vi "Destroy Class ObjData.vi"(8 "error in (no error)":errorcluster, 11 "Motor Controller in":refnum<class "Motor Controller.lvclass">) -> (0 "error out":errorcluster, 3 "Motor Controller out":refnum<class "Motor Controller.lvclass">)   [LabVIEW 2022 SP3, in "Motor Controller.lvclass"]
uses:
  Motor Controller.lvclass
  Motor Controller.lvclass/Motor Controller.ctl
panel:
  out "ObjData Variant":variant
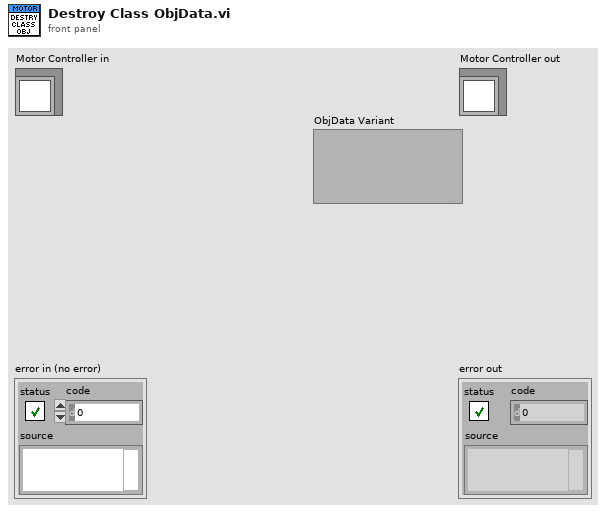
[diagram p1: front panel]
types:
  T1 = typedef "Motor Controller.lvclass/Private Data.ctl" = cluster{"UserEvents":T2, "All Dependencies":cluster{"Class References":refnum<class>[], "Class Names":string[]}, "Status":T3}
  T2 = typedef "Motor Controller.lvclass/UserEvents.ctl" = cluster{"API Incoming Event":refnum<user-event>, "API Executed Event":refnum<user-event>, "API Return Event":refnum<user-event>, "Status Changed Event":refnum<user-event>, "StopEvent":refnum<user-event>}
  T3 = typedef "Motor Controller.lvclass/Status.ctl" = cluster{"Motor Controller Config Data":T4, "Motor Controller Data":cluster{"Enabled?":bool}, "Stage Move":T5, "Stage Busy?":bool}
  T4 = typedef "Motor Controller.lvclass/Motor Controller Config Data.ctl" = cluster{"Motor IP Addresss":string, "Current Position":i32, "Pulse_Per_mm":i32, "PrePrint":dbl[], "Load Position_mm":i32, "Laminate Position_mm":i32}
  T5 = typedef "Motor Controller.lvclass/Stage Move Data.ctl" = cluster{"Current Step":string, "Move Data":T6[]}
  T6 = typedef "Motor Controller.lvclass/Batch Index Speed Data.ctl" = cluster{"Batch & Cycle":string, "Move":cluster{"Index_mm":i32, "Speed_mm_s":i32}, "Status":T7}
  T7 = typedef "Motor Controller.lvclass/Move Status.ctl" = enum16{"Pending", "In Progress", "Completed"}
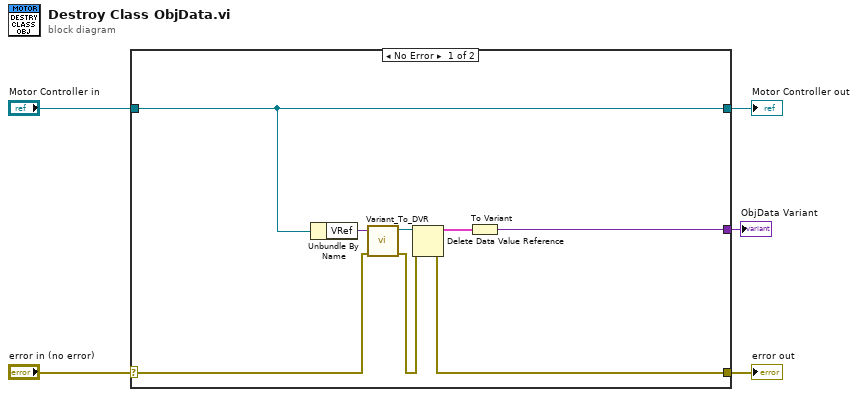
[diagram p0: block diagram]
diagram:
  n1 = case shown="No Error" "error in (no error)" {
    selector: "error in (no error)" -> [w9 w15]
    tunnel: [w7 w15] -> w4
    tunnel: [w12 w14] -> w2
    tunnel: "Motor Controller in" -> [w12 w14]
    tunnel: [w6 _] -> w1
    frame No Error {
      n2 = Unbundle By Name(w12) -> ("VRef"=w11:variant)
      n3 = call "Variant_To_DVR.vi"("error in (no error)"=w9, "Variant"=w11) -> ("error out"=w8:errorcluster, "DVR"=w10:refnum<data-value>)  [unwired: 8 in]
      n4 = Delete Data Value Reference(data value reference=w10, error in=w8) -> (data value=w13:T1, error out=w7:errorcluster)
      n5 = To Variant(anything=w13) -> (Variant=w6:variant)
    }
    frame Error {
    }
  }
  "error out" <- w4
  "Motor Controller out" <- w2
  "ObjData Variant" <- w1
